vi "ExSubCascadeTTLout.vi"(2 "error in (no error)":errorcluster, 3 "Value to Output":u32, 4 "Camera Handle":u32) -> (0 "error out":errorcluster, 1 "Camera Handle":u32)   [LabVIEW 2010]
panel:
  # "ExSubCascadeTTLout - output value (0-255)\nout the TTL lines of Cascade (8 lines)."
  # "value to put out ttl lines (0-255)"
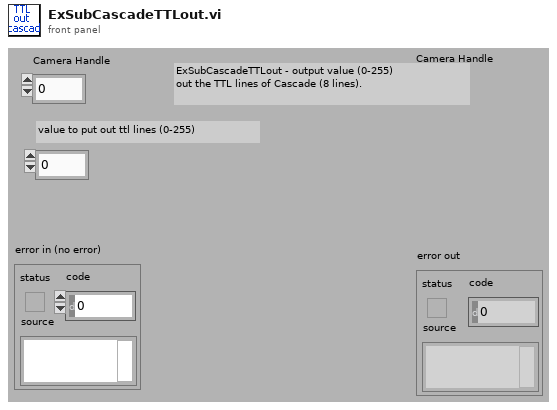
[diagram p1: front panel]
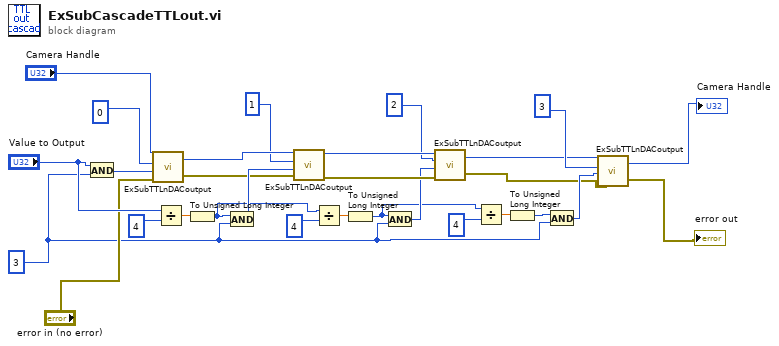
[diagram p0: block diagram]
diagram:
  w8 = 3
  n1 = And(x="Value to Output", y=w8) -> (x .and. y?=w27:u32)
  n2 = call "ExSubTTLnDACoutput.vi"("error in (no error)"="error in (no error)", "Value to Output"=w27, "Port"=0, "Camera Handle"="Camera Handle") -> ("error out"=w20:errorcluster, "Camera Handle"=w26:u32)
  n3 = Divide(x="Value to Output", y=4) -> (x/y=w22:dbl)
  n4 = To Unsigned Long Integer(number=w22) -> (unsigned 32bit integer=w16:u32)
  n5 = And(x=w16, y=w8) -> (x .and. y?=w21:u32)
  n6 = call "ExSubTTLnDACoutput.vi"("error in (no error)"=w20, "Value to Output"=w21, "Port"=1, "Camera Handle"=w26) -> ("error out"=w14:errorcluster, "Camera Handle"=w15:u32)
  n7 = Divide(x=w16, y=4) -> (x/y=w17:dbl)
  n8 = To Unsigned Long Integer(number=w17) -> (unsigned 32bit integer=w7:u32)
  n9 = And(x=w7, y=w8) -> (x .and. y?=w13:u32)
  n10 = call "ExSubTTLnDACoutput.vi"("error in (no error)"=w14, "Value to Output"=w13, "Port"=2, "Camera Handle"=w15) -> ("error out"=w3:errorcluster, "Camera Handle"=w4:u32)
  n11 = Divide(x=w7, y=4) -> (x/y=w9:dbl)
  n12 = To Unsigned Long Integer(number=w9) -> (unsigned 32bit integer=w10:u32)
  n13 = And(x=w10, y=w8) -> (x .and. y?=w6:u32)
  n14 = call "ExSubTTLnDACoutput.vi"("error in (no error)"=w3, "Value to Output"=w6, "Port"=3, "Camera Handle"=w4) -> ("error out"=→"error out":errorcluster, "Camera Handle"=→"Camera Handle":u32)
